vi "Post-Build Action.vi"(5 "Files Generated by Build":path[](array[path]) caption="通过生成创建的文件", 6 "Top Level/Always Included VIs":path[](array[path]) caption="顶层/始终包括VI", 7 "Destination Path":path caption="目标路径", 8 "error in (no error)":errorcluster caption="错误输入（无错误）", 9 "Target Name":string caption="终端名称", 10 "Build Specification Name":string caption="程序生成规范名称", 11 "Project Path":path caption="项目路径") -> (0 "error out":errorcluster caption="错误输出")   [LabVIEW 2019]
uses:
  <userlib>/_OpenG.lib/lvzip/lvzip.llb/ZLIB Open ZIP Mode__ogtk.ctl
  <vilib>/AppBuilder/AB_API_Simple/Get Build Specification Version (path).vi
  <vilib>/Utility/config.llb/Write Key (String).vi
  <vilib>/AppBuilder/AB_API_Simple/NI_App_Builder_API.lvlib
  <vilib>/Utility/config.llb/NI_LVConfig.lvlib
panel:
  out "提示信息":string="正在发布更新至服务器……"
  out "滑动杆":u8(slide) scale=0.0..100.0
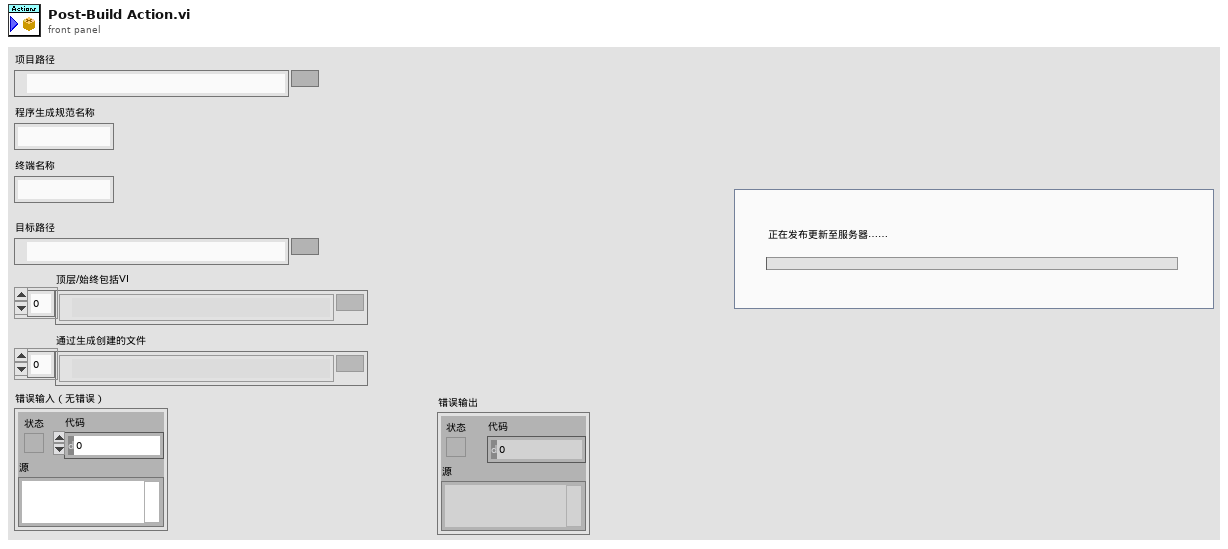
[diagram p1: front panel]
types:
  T1 = typedef "ZLIB Open ZIP Mode__ogtk.ctl" = enum16{"create new", "append to end", "append to archive"}
  T2 = typedef "NI_App_Builder_API.lvlib/Build Specification Version.ctl" = cluster{"Major":u16, "Minor":u16, "Fix":u16, "Build":u16}
  T3 = typedef "NI_LVConfig.lvlib/Config Data RefNum.ctl" = refnum<k1>
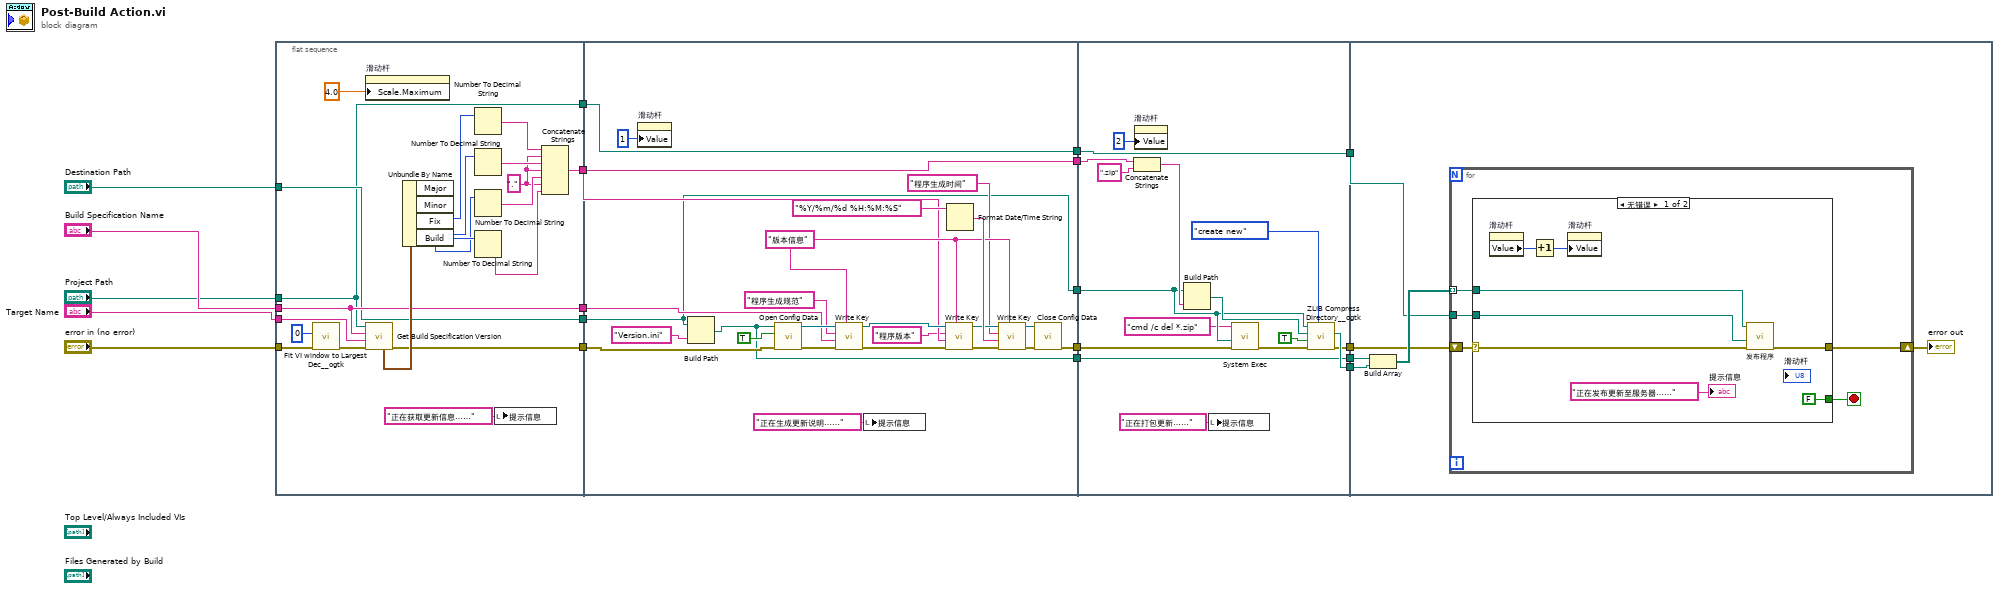
[diagram p0: block diagram]
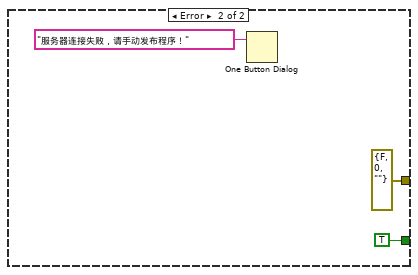
[diagram p2: hidden frame]
diagram:
  n1 = flat-sequence {
    tunnel: "Build Specification Name" -> [w29]
    tunnel: [w28] -> w12
    tunnel: [w26] -> w11
    tunnel: [w29] -> w10
    tunnel: [w27] -> w9
    tunnel: "Target Name" -> [w30]
    tunnel: "Project Path" -> [w22]
    tunnel: "Destination Path" -> [w26]
    tunnel: "error in (no error)" -> [w25]
    tunnel: [w22] -> w5
    tunnel: [w53] -> w18
    tunnel: [w48] -> w17
    tunnel: [w45] -> w16
    tunnel: [w44] -> w13
    tunnel: w12 -> [w53]
    tunnel: w11 -> [w48]
    tunnel: w10 -> [w51]
    tunnel: w9 -> [w47]
    tunnel: w5 -> [w43]
    tunnel: [w43] -> w4
    tunnel: [w72] -> w19
    tunnel: w18 -> [w80]
    tunnel: w17 -> [w75]
    tunnel: w16 -> [w71]
    tunnel: [w70] -> w14
    tunnel: w13 -> [w70]
    tunnel: w4 -> [w69]
    tunnel: [w69] -> w3
    tunnel: [w68] -> w1
    tunnel: w19 -> [w85]
    tunnel: w14 -> [w84]
    tunnel: w3 -> [w83]
    tunnel: w1 -> [w82]
    frame #0 {
      w31 = "." ("字符串")
      n2 = call <userlib>:"Fit VI window to Largest Dec__ogtk.vi"("error in (no error)"=w25, "border spacing (2 px)"=0) -> ("error out"=w23:errorcluster)  [unwired: 4 in, 1 out]
      n3 = property on="滑动杆" class="Slide (严格)"("Scale.Maximum"=4.0 ("标尺.范围:最大值")) -> ()  [unwired: 2 in, 2 out]
      n4 = call-poly <vilib>:"Get Build Specification Version.vi"("error in (no error)"=w23, "Name of target (My Computer)"=w30, "Name of build specification"=w29, "Path to project"=w22) -> ("error out"=w27:errorcluster, "Build Specification Version"=w32:T2)  [unwired: 6 in]
      n5 = Unbundle By Name(w32) -> ("Major"=w33:u16, "Minor"=w34:u16, "Fix"=w35:u16, "Build"=w36:u16)
      n6 = Number To Decimal String(number=w33) -> (decimal integer string=w37:string)  [unwired: 1 in]
      n7 = Number To Decimal String(number=w34) -> (decimal integer string=w38:string)  [unwired: 1 in]
      n8 = Number To Decimal String(number=w35) -> (decimal integer string=w39:string)  [unwired: 1 in]
      n9 = Number To Decimal String(number=w36) -> (decimal integer string=w40:string)  [unwired: 1 in]
      n10 = local write "提示信息"("正在获取更新信息……" ("提示信息")) -> ()
      n11 = Concatenate Strings(w37, w31, w38, w31, w39, w31, w40) -> (w28:string)
    }
    frame #1 {
      w55 = "版本信息" ("section")
      n12 = property on="滑动杆" class="Slide (严格)"("Value"=u8 1 ("滑动杆")) -> ()  [unwired: 2 in, 2 out]
      n13 = Build Path(base path=w48, name or relative path="Version.ini" ("名称或相对路径")) -> (appended path=w44:path)
      n14 = call <vilib>:"Open Config Data.vi"("error in (no error)"=w47, "create file if necessary (T)"=TRUE, "configuration file path"=w44) -> ("error out"=w61:errorcluster, "refnum"=w57:T3)  [unwired: 6 in, 1 out]
      n15 = call-poly <vilib>:"Write Key.vi"("section"=w55, "error in (no error)"=w61, "value"=w51, "key"="程序生成规范", "refnum"=w57) -> ("error out"=w62:errorcluster, "refnum out"=w58:T3)  [unwired: 4 in, 1 out]
      n16 = local write "提示信息"("正在生成更新说明……" ("提示信息")) -> ()
      n17 = call-poly <vilib>:"Write Key.vi"("section"=w55, "error in (no error)"=w62, "value"=w53, "key"="程序版本", "refnum"=w58) -> ("error out"=w63:errorcluster, "refnum out"=w59:T3)  [unwired: 4 in, 1 out]
      n18 = Format Date/Time String(time format string (%c)="%Y/%m/%d %H:%M:%S" ("时间格式字符串(%c)")) -> (date/time string=w60:string)  [unwired: 2 in]
      n19 = call-poly <vilib>:"Write Key.vi"("section"=w55, "error in (no error)"=w63, "value"=w60, "key"="程序生成时间", "refnum"=w59) -> ("error out"=w65:errorcluster, "refnum out"=w64:T3)  [unwired: 4 in, 1 out]
      n20 = call <vilib>:"Close Config Data.vi"("error in (no error)"=w65, "refnum"=w64) -> ("error out"=w45:errorcluster)  [unwired: 8 in, 1 out]
    }
    frame #2 {
      n21 = Concatenate Strings(w80, ".zip" ("字符串")) -> (w81:string)
      n22 = property on="滑动杆" class="Slide (严格)"("Value"=u8 2 ("滑动杆")) -> ()  [unwired: 2 in, 2 out]
      n23 = Build Path(base path=w75, name or relative path=w81) -> (appended path=w76:path)
      n24 = local write "提示信息"("正在打包更新……" ("提示信息")) -> ()
      n25 = call <vilib>:"System Exec.vi"("error in (no error)"=w71, "working directory"=w75, "command line"="cmd /c del *.zip") -> ("error out"=w73:errorcluster)  [unwired: 5 in, 3 out]
      n26 = call <userlib>:"ZLIB Compress Directory__ogtk.vi"("append (create new)"=ZLIB_Open_ZIP_Mode__ogtk."create new", "error in (no error)"=w73, "include subdirectories (F)"=TRUE, "archive name (root directory with .zip ending)"=w76, "root directory (file dialog)"=w75) -> ("error out"=w68:errorcluster, "archive name out"=w72:path)  [unwired: 4 in, 1 out]
    }
    frame #3 {
      n27 = Build Array(w84, w85) -> (w87:path[])
      n28 = for {
        tunnel: w87 -> [w92] mode=indexing
        shift-right: [w91] -> w86
        shift-left: w82 -> [w90]
        tunnel: w83 -> [w88]
        stop <- w89 stop-if-true
        n29 = case shown="无错误" w90 {
          selector: w90 -> [w94 _]
          tunnel: w92 -> [w100 _]
          tunnel: [w99 errorcluster {"status"=FALSE, "code"=0, "source"=""} ("error out")] -> w91
          tunnel: [FALSE TRUE] -> w89
          tunnel: w88 -> [w97 _]
          frame No Error {
            n30 = property on="滑动杆" class="Slide (严格)"() -> ("Value"=w95:u8)  [unwired: 2 in, 2 out]
            n31 = Increment(x=w95) -> (x+1=w96:u8)
            n32 = property on="滑动杆" class="Slide (严格)"("Value"=w96) -> ()  [unwired: 2 in, 2 out]
            n33 = call "发布程序.vi"("error in (no error)"=w94, "项目路径"=w97, "local path"=w100) -> ("error out"=w99:errorcluster)  [unwired: 8 in]
            "提示信息" <- "正在发布更新至服务器……" ("格式字符串")
          }
          frame Error {
            n34 = One Button Dialog(message="服务器连接失败，请手动发布程序！" ("格式字符串")) -> ()  [unwired: 1 in, 1 out]
          }
        }
      }
      "error out" <- w86
    }
  }
